vi "generate system parameters.vi"(8 "error in (no error)":errorcluster, 9 "M-PSK":i32=4, 11 "samples per symbol":i32=16) -> (0 "error out":errorcluster, 3 "system parameters":T1 {"symbol map" format="%.3f"})   [LabVIEW 2011]
uses:
  <vilib>/addons/Modulation/niDMT.lvlib
  <vilib>/addons/Modulation/niAMT.lvlib
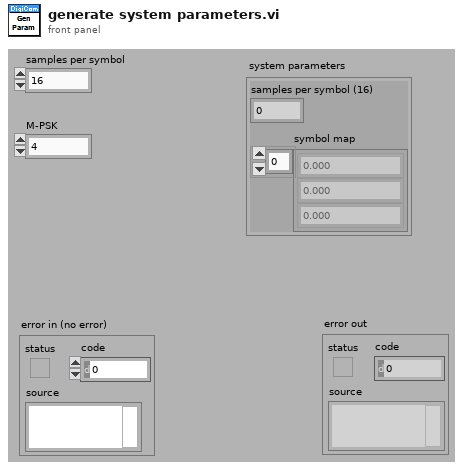
[diagram p1: front panel]
types:
  T1 = cluster{"samples per symbol (16)":i32, "symbol map":cdb[]}
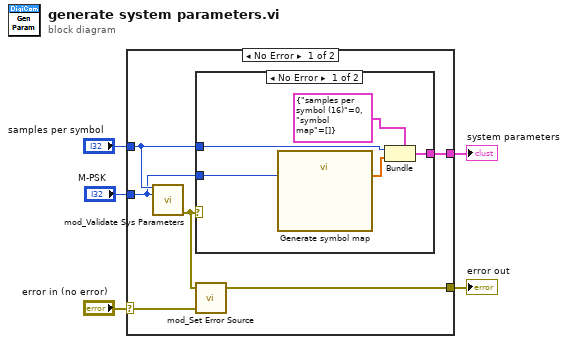
[diagram p0: block diagram]
diagram:
  n1 = case shown="No Error" "error in (no error)" {
    selector: "error in (no error)" -> [w9 w17]
    tunnel: "samples per symbol" -> [w8 _]
    tunnel: [w11 _] -> w1
    tunnel: "M-PSK" -> [w7 _]
    tunnel: [w10 w17] -> w3
    frame No Error {
      n2 = call <vilib>:"mod_Validate Sys Parameters.vi"("samples per symbol"=w8, "M-ary"=w7) -> ("error out"=w6:errorcluster)  [unwired: 13 out]
      n3 = case shown="No Error" w6 {
        tunnel: [w16 _] -> w11
        tunnel: w7 -> [w12 _]
        tunnel: w8 -> [w15 _]
        frame No Error {
          n4 = call "Generate symbol map.vi"("M"=w12) -> ("symbol map"=w14:cdb[])  [unwired: 10 in]
          n5 = Bundle(cluster=T1 {"samples per symbol (16)"=0, "symbol map"=[]} ("PSK system parameters 3"), "samples per symbol (16)"=w15, "symbol map"=w14) -> (w16:T1)
        }
        frame Error {
        }
      }
      n6 = call <vilib>:"mod_Set Error Source.vi"("initial error in (no error)"=w9, "final error in (no error)"=w6) -> ("error out"=w10:errorcluster)  [unwired: 3 out]
    }
    frame Error {
    }
  }
  "system parameters" <- w1
  "error out" <- w3
